vi "PH_Timing.Action SetPU-GD.vi"(0 "i ref in":refnum<vi>, 2 "PU":T1, 5 "error in (no error)":errorcluster) -> (14 "i ref out":refnum<vi>, 19 "error out":errorcluster)   [LabVIEW 2014, in "PH_Timing.lvlib"]
doc: "Within this VI the channel configuration is set if the related GD Generator is linked."
uses:
  PH_Timing.lvlib
  PH_Basics/PH_PP_Common/PH_PP_Common.PUs.ctl
  PH_Basics/PH_PP_Common/PH_PP_Common.lvlib
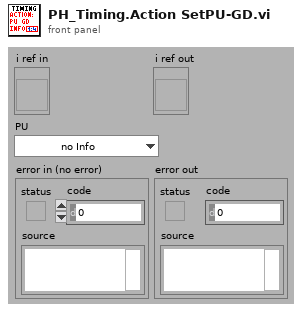
[diagram p1: front panel]
types:
  T1 = typedef "PH_PP_Common.lvlib/PH_PP_Common.PUs.ctl" = enum16{"no Info", "PA-19mm-1", "PA-19mm-2", "PA-45mm-PILC", "PA-45mm-MAIN", "MA-PU-1", "MA-PU-2", "MA-PU-3", "MA-PU-4", "MA-PU-5", "MA-PU-6", "MA-FR", "MA-PILC", "PA-45mm-DP"}
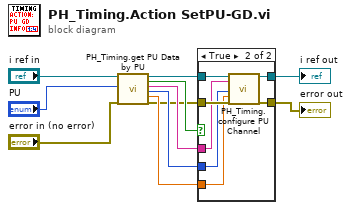
[diagram p0: block diagram]
diagram:
  n1 = call "PH_Timing.get PU Data by PU.vi"("VI in"="i ref in", "PU"="PU", "error in (no error)"="error in (no error)") -> ("VI out"=w2:refnum<vi>, "GD linked?"=w4:bool, "GD Name"=w6:string, "CH"=w5:i32, "Delay"=w3:dbl, "error out"=w1:errorcluster)  [unwired: 9 in, 2 out]
  n2 = case shown="True" w4 {
    tunnel: w1 -> [w12 w20]
    tunnel: w2 -> [w13 w19]
    tunnel: [w12 w18] -> w9
    tunnel: [w13 w17] -> w8
    tunnel: w6 -> [_ w16]
    tunnel: w5 -> [_ w15]
    tunnel: w3 -> [_ w14]
    frame False {
    }
    frame True {
      n3 = call "PH_Timing.configure PU Channel.vi"("i ref in"=w19, "GateGen Instance"=w16, "Channel"=w15, "Delay"=w14, "error in"=w20) -> ("i ref out"=w17:refnum<vi>, "error out"=w18:errorcluster)  [unwired: 13 in]
    }
  }
  "error out" <- w9
  "i ref out" <- w8
